vi "SUB CWT.vi"(4 "f to sigma ratio":dbl=4.0 format="%#_15g", 5 "normalization":u16(ring) items=["Energy", "Amplitude"], 6 "user defined scales":dbl[](array[numeric]), 7 "time steps":i32=-1, 8 "error in (no error)":errorcluster, 9 "scale sampling method":u16(ring) items=["Even frequency", "Even scale"], 10 "scales":i32=128 min=1, 11 "signal":waveform(dbl)={"t0"=timestamp(0 s since 1904-01-01), "dt"=0.0, "Y"=[]}) -> (0 "error out":errorcluster, 2 "scale info":variant, 3 "AWT coef":cdb[][](array[numeric]))   [LabVIEW 2017]
uses:
  <vilib>/addons/_Advanced Signal Processing/NI_AdvSigProcWA.lvlib
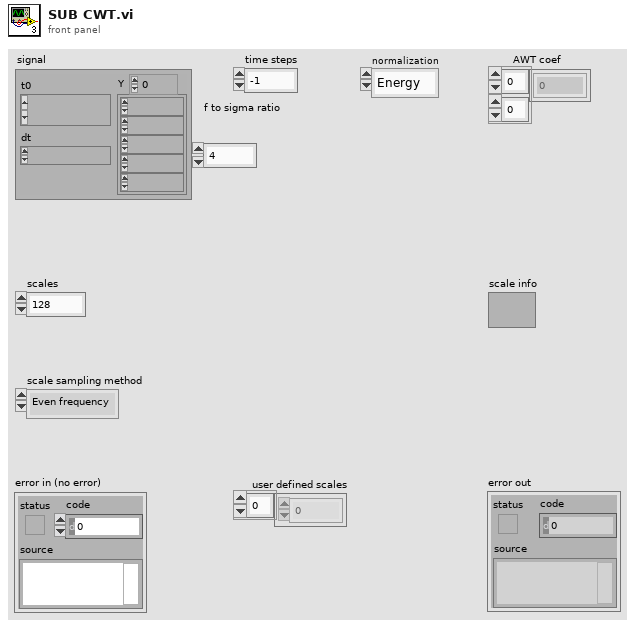
[diagram p1: front panel]
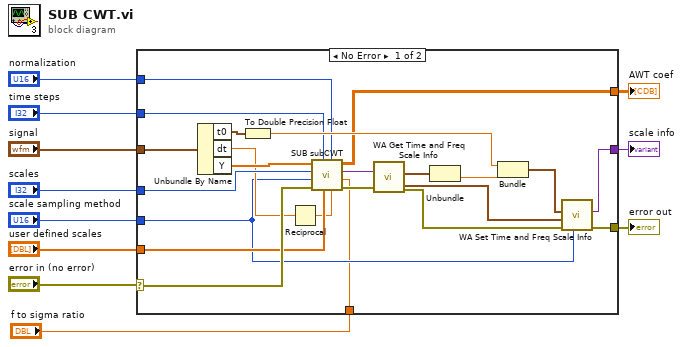
[diagram p0: block diagram]
diagram:
  n1 = case shown="No Error" "error in (no error)" {
    selector: "error in (no error)" -> [w32 w35]
    tunnel: [w14 w35] -> w10
    tunnel: "normalization" -> [w30 _]
    tunnel: "time steps" -> [w29 _]
    tunnel: "signal" -> [w28 _]
    tunnel: "scales" -> [w27 _]
    tunnel: "scale sampling method" -> [w15 _]
    tunnel: "user defined scales" -> [w22 _]
    tunnel: [w21 _] -> w3
    tunnel: [w13 _] -> w2
    tunnel: "f to sigma ratio" -> [w12 _]
    frame No Error {
      n2 = Unbundle By Name(w28) -> ("t0"=w34:timestamp, "dt"=w18:dbl, "Y"=w33:dbl[])
      n3 = To Double Precision Float(number=w34) -> (double precision float=w31:dbl)
      n4 = Reciprocal(x=w18) -> (1/x=w17:dbl)
      n5 = call "SUB subCWT.vi"("f to sigma ratio"=w12, "sampling rate"=w17, "normalization"=w30, "user defined scales"=w22, "time steps"=w29, "error in (no error)"=w32, "scale sampling method"=w15, "scales"=w27, "signal"=w33) -> ("error out"=w23:errorcluster, "scale info"=w25:variant, "AWT coef"=w21:cdb[][])
      n6 = call <vilib>:"WA Get Time and Freq Scale Info.vi"("error in (no error)"=w23, "scale info"=w25) -> ("error out"=w19:errorcluster, "frequency info"=w16:cluster{"offset":dbl, "multiplier":dbl}, "time info"=w24:cluster{"offset":dbl, "multiplier":dbl})  [unwired: 7 out]
      n7 = Unbundle(w24) -> ("multiplier"=w20:dbl)  [unwired: 1 out]
      n8 = Bundle(w31, "multiplier"=w20) -> (w26:cluster{dbl, "multiplier":dbl})  [unwired: 1 out]
      n9 = call <vilib>:"WA Set Time and Freq Scale Info.vi"("scale sampling method"=w15, "error in (no error)"=w19, "frequency info"=w16, "time info"=w26) -> ("error out"=w14:errorcluster, "scale info"=w13:variant)  [unwired: 6 out]
    }
    frame Error {
    }
  }
  "error out" <- w10
  "AWT coef" <- w3
  "scale info" <- w2
